vi "Timer_Stop.vi"(8 "error in (no error)":errorcluster, 10 "Is Paused?":bool=TRUE, 11 "Timer Data Reference (in)":refnum<data-value>) -> (0 "error out":errorcluster, 3 "Timer Data Reference (out)":refnum<data-value>)   [LabVIEW 2024]
doc: "Stops the Timer DVR\n\n--------\nPaulo Rossi\nprossi@aurumautomation.ca\n©2024 Aurum Automation Inc.\nOpen-Sourced per GNU GPL v3\n\nYou should have received a copy of the GNU General Public License along with this program. If not, see <https://www.gnu.org/licenses/>."
uses:
  Timer_Data.ctl
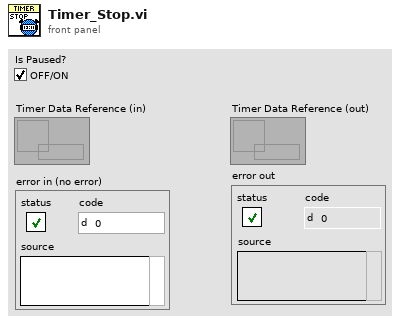
[diagram p1: front panel]
types:
  T1 = typedef "Timer_Data.ctl" = cluster{"Starting Time":dbl, "Time Elapsed (s)":dbl, "Is Time Elapsed?":bool, "Target Time (s)":dbl, "Pause Start Time":dbl, "Pause Elapsed Time":dbl, "Is Paused?":bool, "Cumulative Paused Time":dbl}
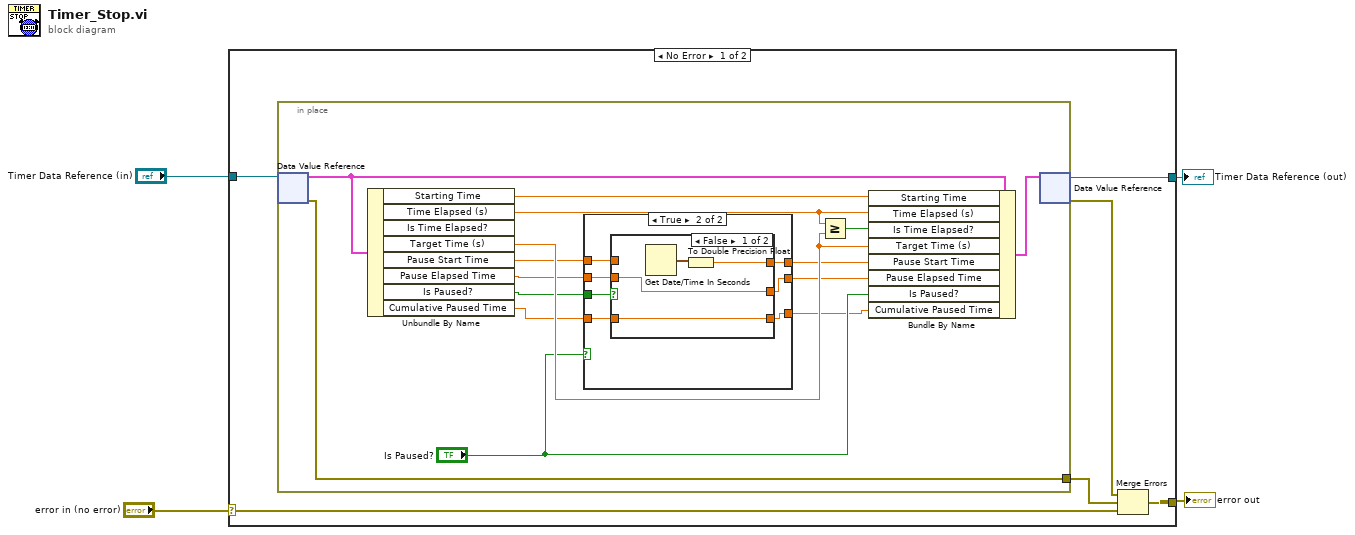
[diagram p0: block diagram]
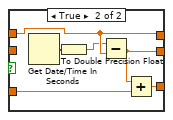
[diagram p3: hidden frame]
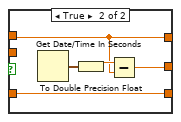
[diagram p4: hidden frame]
diagram:
  n1 = case shown="No Error" "error in (no error)" {
    selector: "error in (no error)" -> [w5 w59]
    tunnel: [w8 w59] -> w3
    tunnel: "Timer Data Reference (in)" -> [w10 w58]
    tunnel: [w9 w58] -> w1
    frame No Error {
      n2 = in-place {
        in-place-border: [w24] -> w6
        n3 = in-place-dvr #1(w10) -> (w23:T1, w24:errorcluster)
        n4 = Unbundle By Name(w23) -> ("Starting Time"=w22:dbl, "Time Elapsed (s)"=w16:dbl, "Target Time (s)"=w20:dbl, "Pause Start Time"=w17:dbl, "Pause Elapsed Time"=w19:dbl, "Is Paused?"=w15:bool, "Cumulative Paused Time"=w11:dbl)  [unwired: 1 out]
        n5 = case shown="True" "Is Paused?" {
          tunnel: w19 -> [w29 w44]
          tunnel: [w31 w48] -> w18
          tunnel: w17 -> [w32 w47]
          tunnel: w15 -> [w30 w46]
          tunnel: [w28 w45] -> w13
          tunnel: [w27 w42] -> w12
          tunnel: w11 -> [w26 w43]
          frame False {
            n6 = case shown="False" w30 {
              tunnel: [w35 w40] -> w31
              tunnel: w32 -> [w35 w40]
              tunnel: [w34 w38] -> w28
              tunnel: w29 -> [w34 _]
              tunnel: [w33 w37] -> w27
              tunnel: w26 -> [w33 w36]
              frame False {
              }
              frame True {
                n7 = Get Date/Time In Seconds() -> (seconds since 1Jan1904=w41:timestamp)
                n8 = To Double Precision Float(number=w41) -> (double precision float=w39:dbl)
                n9 = Subtract(x=w39, y=w40) -> (x-y=w38:dbl)
                n10 = Add(x=w38, y=w36) -> (x+y=w37:dbl)
              }
            }
          }
          frame True {
            n11 = case shown="False" w46 {
              tunnel: [w51 w55] -> w48
              tunnel: w47 -> [_ w55]
              tunnel: [w50 w54] -> w45
              tunnel: w44 -> [w50 _]
              tunnel: [w49 w53] -> w42
              tunnel: w43 -> [w49 w53]
              frame False {
                n12 = Get Date/Time In Seconds() -> (seconds since 1Jan1904=w52:timestamp)
                n13 = To Double Precision Float(number=w52) -> (double precision float=w51:dbl)
              }
              frame True {
                n14 = Get Date/Time In Seconds() -> (seconds since 1Jan1904=w57:timestamp)
                n15 = To Double Precision Float(number=w57) -> (double precision float=w56:dbl)
                n16 = Subtract(x=w56, y=w55) -> (x-y=w54:dbl)
              }
            }
          }
        }
        n17 = Greater Or Equal?(x=w16, y=w20) -> (x >= y?=w21:bool)
        n18 = Bundle By Name(cluster=w23, "Starting Time"=w22, "Time Elapsed (s)"=w16, "Is Time Elapsed?"=w21, "Target Time (s)"=w20, "Pause Start Time"=w18, "Pause Elapsed Time"=w13, "Is Paused?"="Is Paused?", "Cumulative Paused Time"=w12) -> (w25:T1)
        n19 = in-place-dvr #1(w25) -> (w9:refnum<data-value>, w7:errorcluster)
      }
      n20 = Merge Errors(w7, w6, w5) -> (w8:errorcluster)
    }
    frame Error {
    }
  }
  "error out" <- w3
  "Timer Data Reference (out)" <- w1
